vi "Read Lines.vi"(8 "error in (no error)":errorcluster, 11 "ThreePhasePLL configuration in":refnum<class "ThreePhasePLL configuration.lvclass">) -> (0 "error out":errorcluster, 2 "Lines":T1(array[cluster]), 3 "ThreePhasePLL configuration out":refnum<class "ThreePhasePLL configuration.lvclass">)   [LabVIEW 2017, in "ThreePhasePLL configuration.lvclass"]
uses:
  ThreePhasePLL configuration.lvclass
  <vilib>/NI/Tag Bus Module Framework/channel/TBM channel.lvclass
  ThreePhasePLL configuration.lvclass/ThreePhasePLL configuration.ctl
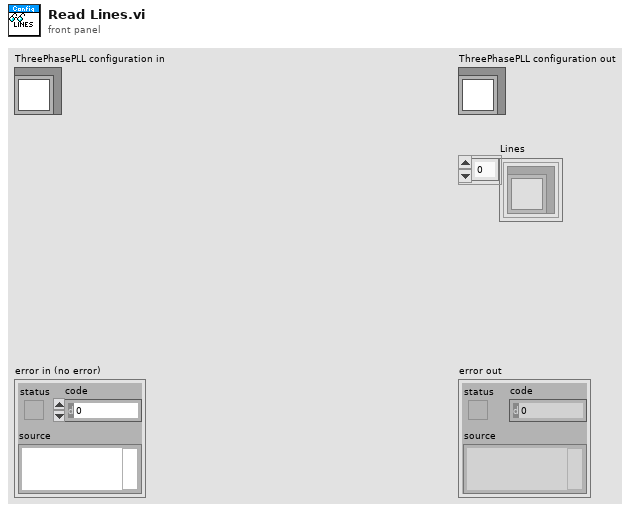
[diagram p1: front panel]
types:
  T1 = cluster{"channel":refnum<class "TBM channel.lvclass">}[]
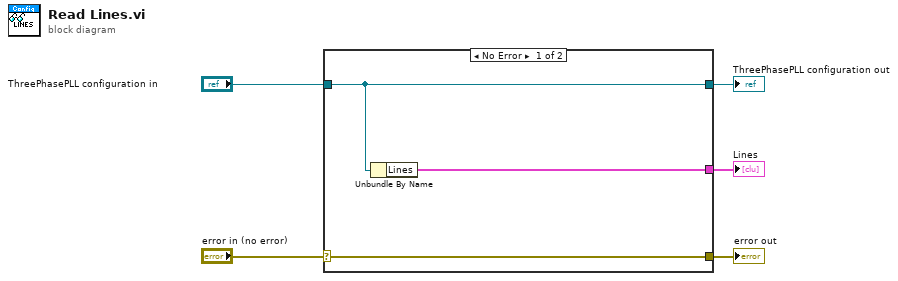
[diagram p0: block diagram]
diagram:
  n1 = case shown="No Error" "error in (no error)" {
    selector: "error in (no error)" -> [w8 w9]
    tunnel: [w8 w9] -> w4
    tunnel: [w7 w10] -> w2
    tunnel: "ThreePhasePLL configuration in" -> [w7 w10]
    tunnel: [w6 _] -> w1
    frame No Error {
      n2 = Unbundle By Name(w7) -> ("Lines"=w6:T1)
    }
    frame Error {
    }
  }
  "error out" <- w4
  "ThreePhasePLL configuration out" <- w2
  "Lines" <- w1
